vi "grabber image display panel.vi"() -> ()   [LabVIEW 2010]
uses:
  internal_queues.ctl
  line_info.ctl
  volume_with_lines.ctl
  volume_info.ctl
  kalman_result_scaled.ctl
  location3D.ctl
  spot location.ctl
  scan_specification_tagResonant.ctl
panel:
  in  "scaling info":T2={" scan settings"={"z resolution (pixels)"=0, "iterations per pixel"=0, "iterations per z-scan (=zres*iterperpixel)"=0, "x resolution (pixels)"=0, "y resolution (pixels)"=0, "number of z-lines per volume"=0, "number of repetitions (volumes)"=0, "Pockels cell voltage (bits)"=0, "Vx center (bits)"=0, "Vy center (bits)"=0, "Vx amplitude (bits)"=0, "Vy amplitude (bits)"=0, "lines to delay between scan start and output"=0, "LSB has acquire control"=FALSE, "Pockels cell bleach voltage"=0}, "scale factors (um/level)"=[0.016, 0.016, 0.00025], "z-feedback range"=2560, "r sphere/sigma"=180.0}
  in  "Queues":T3
  in  "pixel range xy":u8=10
  in  "auto advance?":bool=TRUE
  in  "num spots":u8=1
  in  "spot to set":u8
  out "location constraints":T4(array[cluster])
  in  "spilt ff/fb":bool
  out "XZ view":T5(plugin-control)
  out "ZY view":T5(plugin-control)
  out "XY view":T5(plugin-control)
  out "deltaZ":dbl
  out "pixel sums":cluster{"ch0 sum":u32, "ch1 sum":u32}
  in  "display channels":cluster{"CH0":bool, "CH1":bool}={"CH0"=TRUE, "CH1"=TRUE}
  out "max values from im":T6
  in  "max values":T7={"xy max"={"r max"=-1.0, "g max"=-1.0, "b max"=-1.0}, "xz max"={"r max"=-1.0, "g max"=-1.0, "b max"=-1.0}, "zy max"={"r max"=-1.0, "g max"=-1.0, "b max"=-1.0}}
  in  "turn on displays":bool=TRUE
  in  "xyz order":bool
  in  "stop":bool
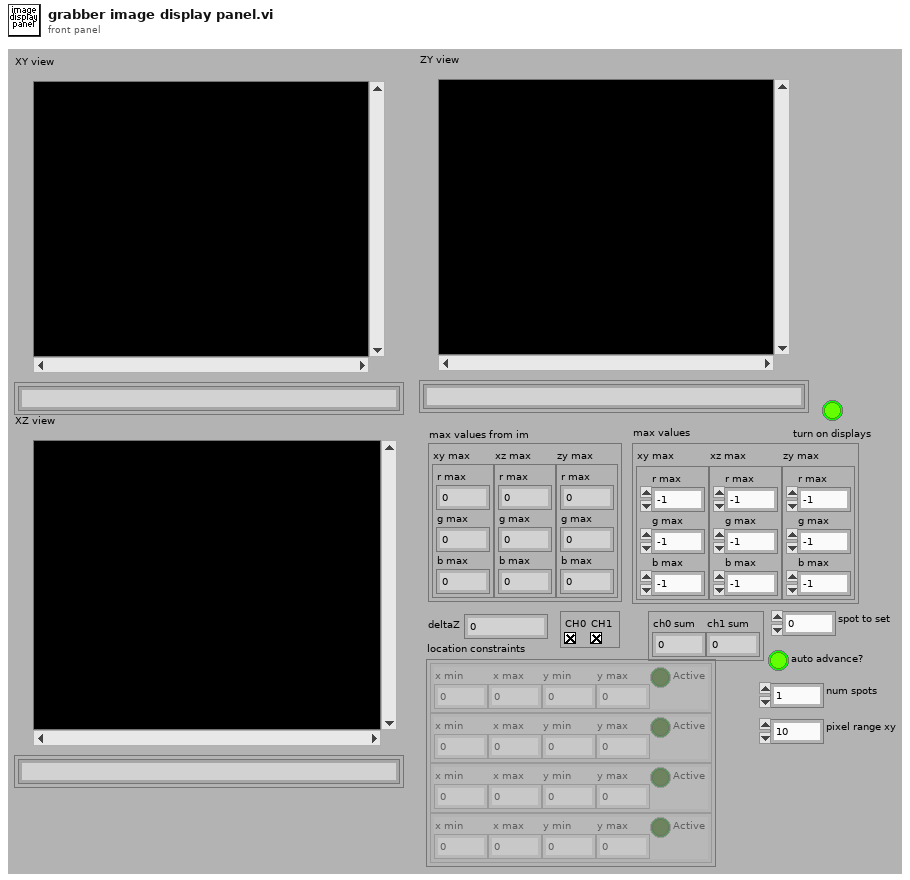
[diagram p1: front panel]
types:
  T1 = typedef "scan_specification_tagResonant.ctl" = cluster{"z resolution (pixels)":u16, "iterations per pixel":u16, "iterations per z-scan (=zres*iterperpixel)":u16, "x resolution (pixels)":u16, "y resolution (pixels)":u16, "number of z-lines per volume":u16, "number of repetitions (volumes)":i32, "Pockels cell voltage (bits)":i16, "Vx center (bits)":i16, "Vy center (bits)":i16, "Vx amplitude (bits)":i16, "Vy amplitude (bits)":i16, "lines to delay between scan start and output":u16, "LSB has acquire control":bool, "Pockels cell bleach voltage":i16}
  T2 = cluster{" scan settings":T1, "scale factors (um/level)":dbl[], "z-feedback range":i16, "r sphere/sigma":dbl}
  T3 = typedef "internal_queues.ctl" = cluster{"volumeQueue":refnum<queue>, "linesWithoutDataQueue":refnum<queue>, "lineQueue":refnum<queue>, "volumesWithLinesQueue":refnum<queue>, "kalmanQueue":refnum<queue>, "completedVolumeQueue":refnum<queue>, "displayVolumeQueue":refnum<queue>, "scanLocationsQueue":refnum<queue>, "kalmanToDisplayPanel":refnum<queue>, "focalPositionQueue":refnum<queue>, "spotPositionsToImagePanel":refnum<queue>}
  T4 = cluster{"x min":i32, "x max":i32, "y min":i32, "y max":i32, "Active":bool}[]
  T5 = typedef "IMAQ Image.ctl" = refnum<image>
  T6 = cluster{"xy max":cluster{"r max":u32, "g max":u32, "b max":u32}, "xz max":cluster{"r max":u32, "g max":u32, "b max":u32}, "zy max":cluster{"r max":u32, "g max":u32, "b max":u32}}
  T7 = cluster{"xy max":cluster{"r max":dbl, "g max":dbl, "b max":dbl}, "xz max":cluster{"r max":dbl, "g max":dbl, "b max":dbl}, "zy max":cluster{"r max":dbl, "g max":dbl, "b max":dbl}}
  T8 = cluster{"x min":i32, "x max":i32, "y min":i32, "y max":i32, "Active":bool}
  T9 = typedef "Image Type" = u32
  T10 = cluster{"New Image":T5, "New Image":T5, "New Image":T5}
  T11 = typedef "spot location.ctl" = cluster{"x (um)":dbl, "y (um)":dbl, "z (um)":dbl, "spot number":u8}
  T12 = cluster{"ch0 volume":u32[][][], "ch1 volume":u32[][][], "ff 0+1":u32[][][], "fb 0+1":u32[][][]}
  T13 = cluster{"Rectangle":cluster{"Left":i32, "Top":i32, "Right":i32, "Bottom":i32}, "Rectangle":cluster{"Left":i32, "Top":i32, "Right":i32, "Bottom":i32}, "Rectangle":cluster{"Left":i32, "Top":i32, "Right":i32, "Bottom":i32}}[]
  T14 = cluster{"Image Dst Out":T5, "Image Dst Out":T5, "Image Dst Out":T5}
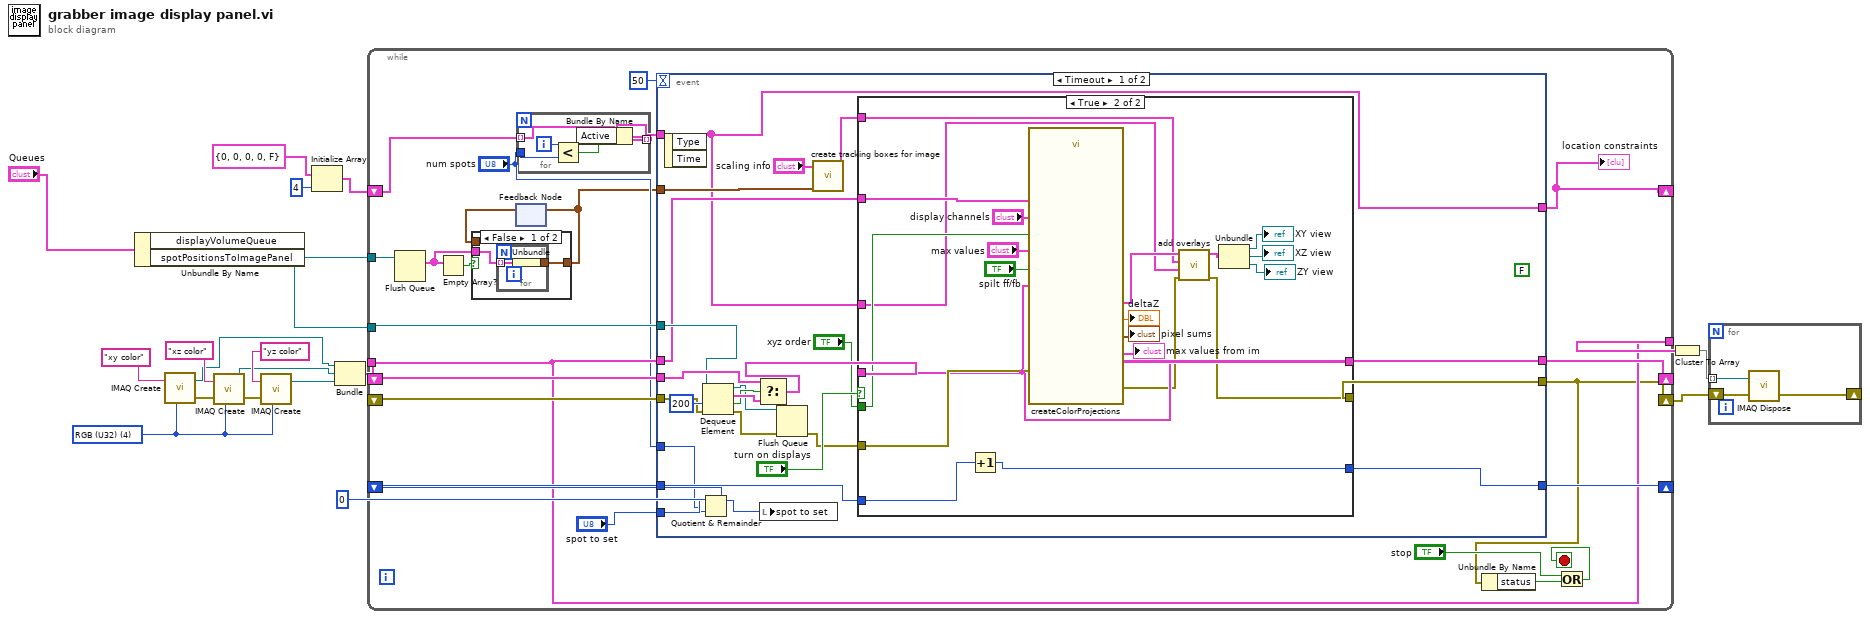
[diagram p0: block diagram]
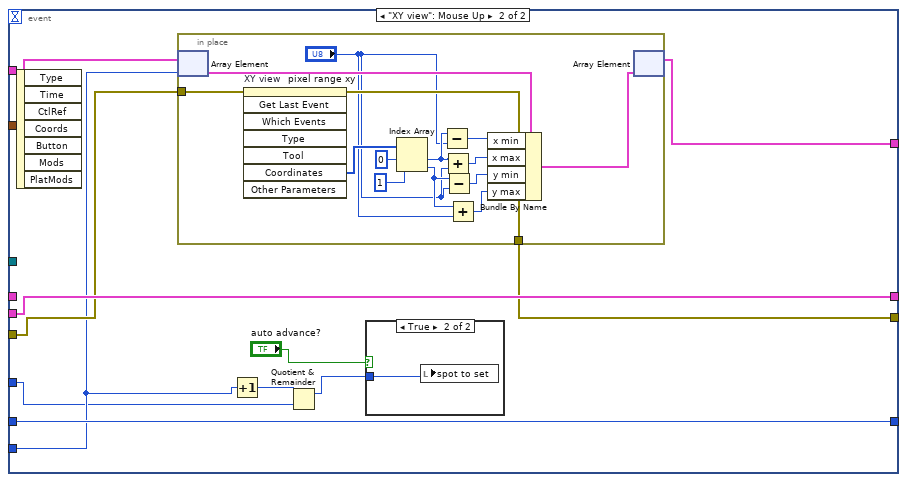
[diagram p4: hidden frame]
diagram:
  w12 = T9 4 items=["Grayscale (U8)", "Grayscale (I16)", "Grayscale (SGL)", "Complex (CSG)", "RGB (U32)", "HSL (U32)", "RGB (U64)", "Grayscale (U16)"] ("Image Type")
  n1 = Unbundle By Name("Queues") -> ("displayVolumeQueue"=w2:refnum<queue>, "spotPositionsToImagePanel"=w1:refnum<queue>)
  n2 = call "IMAQ Create"("Image Name"="xy color", "Image Type"=w12) -> ("New Image"=w15:T5, "error out"=w17:errorcluster)  [unwired: 3 in]
  n3 = call "IMAQ Create"("Image Name"="xz color", "Image Type"=w12, "error in (no error)"=w17) -> ("New Image"=w14:T5, "error out"=w16:errorcluster)  [unwired: 2 in]
  n4 = call "IMAQ Create"("Image Name"="yz color", "Image Type"=w12, "error in (no error)"=w16) -> ("New Image"=w13:T5)  [unwired: 2 in, 1 out]
  n5 = Initialize Array(T8 {"x min"=0, "x max"=0, "y min"=0, "y max"=0, "Active"=FALSE} ("click location"), 4 ("dimension size")) -> (w5:T4)
  n6 = Bundle("New Image"=w15, "New Image"=w14, "New Image"=w13) -> (w11:T10)  [unwired: 1 in]
  n7 = while {
    tunnel: w11 -> [w33]
    shift-right: [w31] -> w7
    shift-left: _ -> [w40]
    shift-right: [w38] -> _
    shift-left: 0 -> [w39]
    shift-right: [w37] -> _
    shift-left: _ -> [w36]
    tunnel: w2 -> [w35]
    tunnel: [w33] -> w9
    shift-right: [w29] -> _
    shift-left: w5 -> [w28]
    tunnel: w1 -> [w21]
    stop <- w41 stop-if-true
    n8 = Flush Queue(queue=w21) -> (remaining elements=w24:cluster{T11[]}[])  [unwired: 1 in, 2 out]
    n9 = Empty Array?(array=w24) -> (empty?=w25:bool)
    n10 = feedback #1() -> (w23:T11[])  [unwired: 1 in]
    n11 = case shown="False" w25 {
      tunnel: w24 -> [w44 _]
      tunnel: [w43 w47] -> w22
      tunnel: w23 -> [_ w47]
      frame False {
        n12 = for {
          tunnel: w44 -> [w46] mode=indexing
          tunnel: [w45] -> w43
          n13 = Unbundle(w46) -> (w45:T11[])
        }
      }
      frame True {
      }
    }
    n14 = feedback-in #1(w22) -> ()
    n15 = for {
      tunnel: w28 -> [w52] mode=indexing
      tunnel: [w49] -> w27 mode=indexing
      tunnel: "num spots" -> [w48]
      i -> [w51]
      n16 = Less?(x=w51, y=w48) -> (x < y?=w50:bool)
      n17 = Bundle By Name(cluster=w52, "Active"=w50) -> (w49:T8)
    }
    n18 = event shown="[0] Timeout" {
      selector: _ -> [_ _]
      dyn-events: _ -> [_ _]
      timeout: 50 -> [_ _]
      tunnel: [w76 w108] -> w31
      tunnel: w40 -> [w74 w109]
      tunnel: w39 -> [w73 w110]
      tunnel: [w72 w110] -> w38
      tunnel: [w71 w111] -> w37
      tunnel: w36 -> [w66 w111]
      tunnel: w35 -> [w62 _]
      tunnel: w33 -> [w60 _]
      tunnel: w27 -> [w53 w107]
      tunnel: [w53 w106] -> w29
      tunnel: "spot to set" -> [w59 w105]
      tunnel: "num spots" -> [w57 w103]
      tunnel: w22 -> [w56 _]
      event Timeout {
        (unwired) FALSE ("auto-update")
        n19 = event-data() -> ()  [unwired: 1 in, 2 out]
        n20 = Quotient & Remainder(x=w59, y=w57) -> (x-y*floor(x/y)=w58:u8)  [unwired: 1 out]
        n21 = Dequeue Element(queue=w62, timeout in ms (-1)=200, error in (no error)=w74) -> (queue out=w63:refnum<queue>, element=w70:T12, timed out?=w69:bool, error out=w65:errorcluster)
        n22 = Select(t=w66, s=w69, f=w70) -> (s? t:f=w67:T12)
        n23 = local write "spot to set"(w58) -> ()
        n24 = Flush Queue(queue=w63, error in (no error)=w65) -> (error out=w64:errorcluster)  [unwired: 2 out]
        n25 = call "create tracking boxes for image.vi"("spot locations"=w56, "scaling info"="scaling info") -> ("Overlay Rectangles"=w55:T13)  [unwired: 9 in]
        n26 = case shown="True" "turn on displays" {
          tunnel: w60 -> [_ w100]
          tunnel: [w79 w86] -> w76
          tunnel: w67 -> [w77 w96]
          tunnel: w64 -> [w79 w99]
          tunnel: w73 -> [w78 w98]
          tunnel: [w78 w97] -> w72
          tunnel: [w77 w96] -> w71
          tunnel: "xyz order" -> [_ w95]
          tunnel: w53 -> [_ w81]
          tunnel: w55 -> [_ w80]
          frame False {
          }
          frame True {
            n27 = Increment(x=w98) -> (x+1=w97:i32)
            n28 = call "createColorProjections.vi"("xyz order"=w95, "max values"="max values", "display channels"="display channels", "error in (no error)"=w99, "spilt ff/fb"="spilt ff/fb", "color ims"=w100, "volumes for display"=w96) -> ("error out"=w87:errorcluster, "deltaZ"=→"deltaZ":dbl, "pixel sums"=→"pixel sums":cluster{"ch0 sum":u32, "ch1 sum":u32}, "color ims out"=w88:T14, "max values from im"=→"max values from im":T6)
            n29 = call "add overlays.vi"("error in (no error)"=w87, "location constraints"=w81, "Overlay Rectangles"=w80, "color ims"=w88) -> ("error out"=w86:errorcluster, "color ims out"=w85:cluster{"xy im":T5, "xz im":T5, "zy im":T5})  [unwired: 6 in]
            n30 = Unbundle(w85) -> ("xy im"=→"XY view":T5, "xz im"=→"XZ view":T5, "zy im"=→"ZY view":T5)
          }
        }
      }
      event "XY view": Mouse Up {
        n31 = event-data() -> ()  [unwired: 1 in, 7 out]
        n32 = in-place {
          in-place-border: w109 -> [w123]
          in-place-border: [w122] -> w108
          n33 = in-place-array #2(w107, w105) -> (w121:T8)
          n34 = invoke on="XY view" class="ImageControl" method="Get Last Event"(error in=w123) -> (error out=w122:errorcluster, "Coordinates"=w126:i32[])  [unwired: 7 in, 6 out]
          n35 = Index Array(array=w126, index #1=0 ("index"), index #2=1 ("index")) -> (element #1=w118:i32, element #2=w117:i32)
          n36 = Subtract(x=w118, y="pixel range xy") -> (x-y=w119:i32)
          n37 = Add(x=w118, y="pixel range xy") -> (x+y=w115:i32)
          n38 = Subtract(x=w117, y="pixel range xy") -> (x-y=w114:i32)
          n39 = Add(x=w117, y="pixel range xy") -> (x+y=w113:i32)
          n40 = Bundle By Name(cluster=w121, "x min"=w119, "x max"=w115, "y min"=w114, "y max"=w113) -> (w120:T8)
          n41 = in-place-array #2(w120) -> (w106:T4)  [unwired: 1 out]
        }
        n42 = Increment(x=w105) -> (x+1=w104:u8)
        n43 = Quotient & Remainder(x=w104, y=w103) -> (x-y*floor(x/y)=w101:u8)  [unwired: 1 out]
        n44 = case shown="True" "auto advance?" {
          tunnel: w101 -> [_ w112]
          frame False {
          }
          frame True {
            n45 = local write "spot to set"(w112) -> ()
          }
        }
      }
    }
    "location constraints" <- w29
    n46 = Unbundle By Name(w31) -> ("status"=w42:bool)
    n47 = Or(x="stop", y=w42) -> (x .or. y?=w41:bool)
  }
  n48 = Cluster To Array(cluster=w9) -> (array=w8:T5[])
  n49 = for {
    tunnel: w8 -> [w129] mode=indexing
    shift-right: [w127] -> _
    shift-left: w7 -> [w128]
    n50 = call "IMAQ Dispose"("Image"=w129, "error in (no error)"=w128) -> ("error out"=w127:errorcluster)  [unwired: 4 in]
  }
